vi "ThreePhasePLL.vi"(0 "Vq":sgl, 1 "PLLgains":T4 {"proportional gain" step=0.125}, 2 "Resources":T1, 3 "PLLrange":T3={"output high (Inf)"=inf, "output low (-Inf)"=-inf}, 5 "dT":sgl, 9 "GridExpectedFreq":sgl, 11 "Phase In":sgl, 12 "reset":bool) -> (4 "gridFrequency":sgl, 10 "PLLactions":T2, 15 "Phase Out":sgl)   [LabVIEW 2017]
uses:
  <vilib>/rvi/Analysis/control/PID/Typedef/niFpgaPID_PIGains.ctl
  <vilib>/rvi/Analysis/control/PID/Typedef/niFpgaPID_OutputRange.ctl
  <vilib>/rvi/Analysis/control/PID/Typedef/niFpgaPID_PIActions.ctl
  Multiplier/Multiplier.lvclass
  Adder/Adder.lvclass
  Subtractor/Subtractor.lvclass
  <vilib>/rvi/Analysis/control/PID/Typedef/niFpgaPID_PIState.ctl
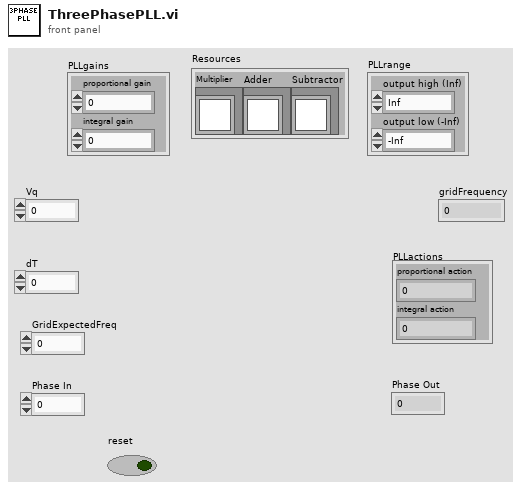
[diagram p1: front panel]
types:
  T1 = cluster{"Multiplier":refnum<class "Multiplier.lvclass">, "Adder":refnum<class "Adder.lvclass">, "Subtractor":refnum<class "Subtractor.lvclass">}
  T2 = typedef "niFpgaPID_PIActions.ctl" = cluster{"proportional action":sgl, "integral action":sgl}
  T3 = typedef "niFpgaPID_OutputRange.ctl" = cluster{"output high (Inf)":sgl, "output low (-Inf)":sgl}
  T4 = typedef "niFpgaPID_PIGains.ctl" = cluster{"proportional gain":sgl, "integral gain":sgl}
  T5 = typedef "niFpgaPID_PIState.ctl" = cluster{"uI(k-1)":sgl, "e(k-1)":sgl, "output (k-1)":sgl}
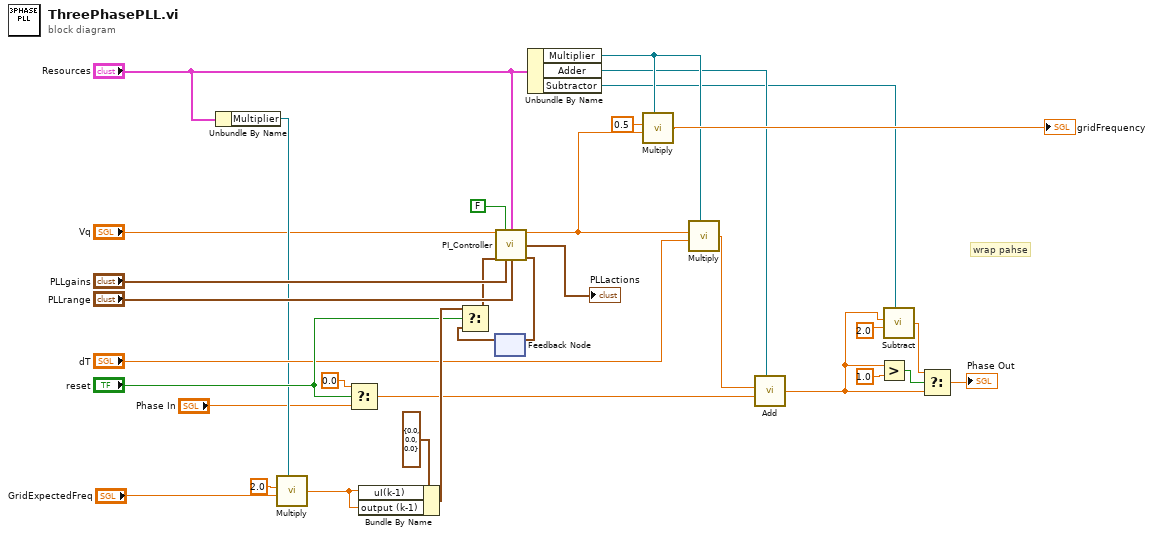
[diagram p0: block diagram]
diagram:
  # "wrap pahse"
  n1 = Unbundle By Name("Resources") -> ("Multiplier"=w11:refnum<class "Multiplier.lvclass">)
  n2 = call-dynamic "Multiply.vi"("x"=sgl 2.0, "y"="GridExpectedFreq", "Multiplier"=w11) -> ("x*y"=w12:sgl)  [unwired: 4 in]
  n3 = Select(t=sgl 0.0, s="reset", f="Phase In") -> (s? t:f=w9:sgl)
  n4 = Bundle By Name(cluster=T5 {"uI(k-1)"=0.0, "e(k-1)"=0.0, "output (k-1)"=0.0} ("state out"), "uI(k-1)"=w12, "output (k-1)"=w12) -> (w25:T5)
  n5 = feedback #1() -> (w24:T5)  [unwired: 1 in]
  n6 = Select(t=w25, s="reset", f=w24) -> (s? t:f=w23:T5)
  n7 = call "PI_Controller.vi"("error"="Vq", "reset? (F)"=FALSE, "Resources"="Resources", "state in"=w23, "gains"="PLLgains", "output range"="PLLrange") -> ("output"=w18:sgl, "actions"=→"PLLactions":T2, "state out"=w33:T5)  [unwired: 6 in, 1 out]
  n8 = feedback-in #1(w33) -> ()
  n9 = Unbundle By Name("Resources") -> ("Multiplier"=w16:refnum<class "Multiplier.lvclass">, "Adder"=w5:refnum<class "Adder.lvclass">, "Subtractor"=w4:refnum<class "Subtractor.lvclass">)
  n10 = call-dynamic "Multiply.vi"("x"=sgl 0.5, "y"=w18, "Multiplier"=w16) -> ("x*y"=→"gridFrequency":sgl)  [unwired: 4 in]
  n11 = call-dynamic "Multiply.vi"("x"=w18, "y"="dT", "Multiplier"=w16) -> ("x*y"=w10:sgl)  [unwired: 4 in]
  n12 = call-dynamic "Add.vi"("x"=w10, "y"=w9, "Adder"=w5) -> ("x+y"=w7:sgl)  [unwired: 4 in]
  n13 = Greater?(x=w7, y=sgl 1.0) -> (0:w29:bool)
  n14 = call-dynamic "Subtract.vi"("x"=w7, "y"=sgl 2.0, "Subtractor"=w4) -> ("x-y"=w6:sgl)  [unwired: 4 in]
  n15 = Select(t=w6, s=w29, f=w7) -> (s? t:f=→"Phase Out":sgl)
